vi "create metadata table.vi"() -> (2 "start time":u32, 3 "lookup table":T1(array[cluster]))   [LabVIEW 2021]
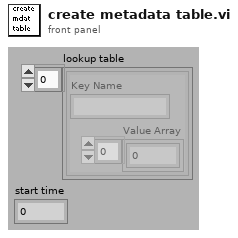
[diagram p1: front panel]
types:
  T1 = cluster{"Key Name":string, "Value Array":dbl[]}[]
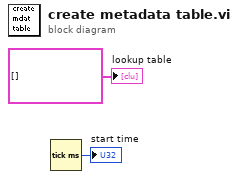
[diagram p0: block diagram]
diagram:
  n1 = Tick Count (ms)() -> (millisecond timer value=→"start time":u32)
  "lookup table" <- T1 [] ("Array")
